vi "String to Array.vi"(0 "Input String":string, 11 "Error In":errorcluster) -> (4 "Array of Strings":string[](array[string]), 15 "Error Out":errorcluster)   [LabVIEW 2023, in "File and Path Operations.lvlib"]
doc: "This VI converts a string into a 1D array, splitting it based on a specified new line delimiter."
uses:
  File and Path Operations.lvlib
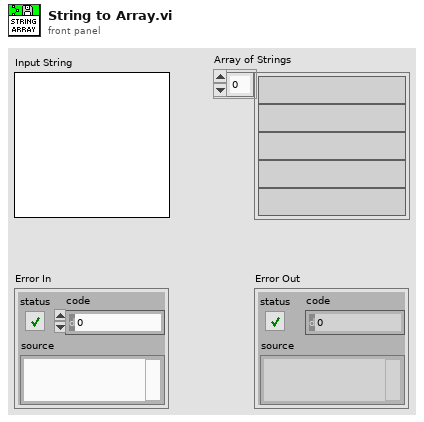
[diagram p1: front panel]
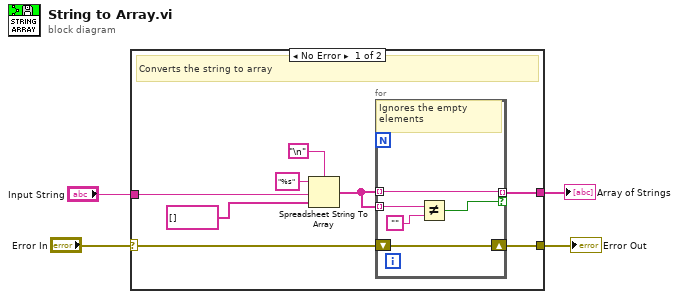
[diagram p0: block diagram]
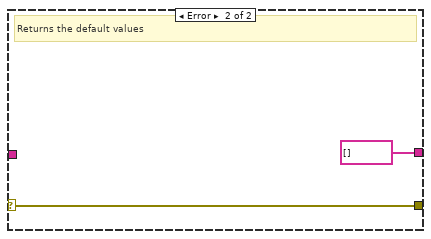
[diagram p2: hidden frame]
diagram:
  n1 = case shown="No Error" "Error In" {
    selector: "Error In" -> [w9 w19]
    tunnel: [w5 string[] []] -> w4
    tunnel: "Input String" -> [w12 _]
    tunnel: [w7 w19] -> w1
    frame No Error {
      # "Converts the string to array"
      n2 = Spreadsheet String To Array(delimiter (Tab)="\n", format string="%s", spreadsheet string=w12, array type (2D Dbl)=string[] []) -> (array=w6:string[])
      n3 = for {
        shift-right: [w17] -> w7
        shift-left: w9 -> [w17]
        tunnel: w6 -> [w16] mode=indexing
        tunnel: [w14] -> w5 mode=indexing if=w13
        tunnel: w6 -> [w14] mode=indexing
        # "Ignores the empty elements"
        n4 = Not Equal?(x=w16, y="") -> (x != y?=w13:bool)
      }
    }
    frame Error {
      # "Returns the default values"
    }
  }
  "Error Out" <- w1
  "Array of Strings" <- w4
